vi "convertRateScanSettingsToString.vi"(8 "error in (no error)":errorcluster, 11 "Model in":refnum<class "Model.lvclass">) -> (0 "error out":errorcluster, 2 "Rate Scan Settings":string, 3 "Model out":refnum<class "Model.lvclass">)   [LabVIEW 2015, in "Model.lvclass"]
uses:
  Model.lvclass
  Model.lvclass/Model.ctl
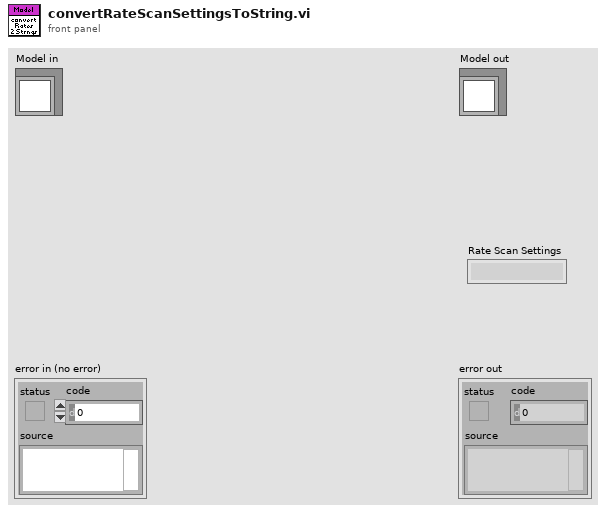
[diagram p1: front panel]
types:
  T1 = typedef "ILCCommon.lvlib/ILCConfiguration.lvlib/Scan Rates.ctl" = enum16{"50", "60", "100", "120", "200", "240", "300", "400", "480", "600", "1200", "2400", "4800"}
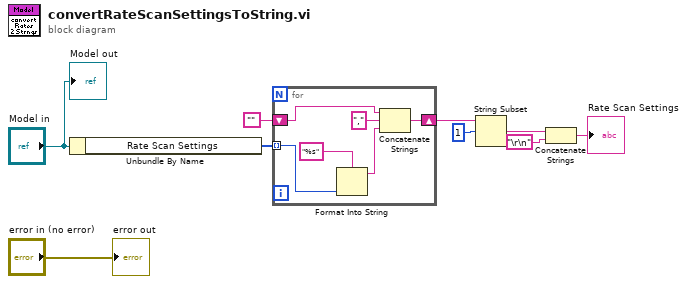
[diagram p0: block diagram]
diagram:
  n1 = Unbundle By Name("Model in") -> ("Rate Scan Settings"=w7:T1[])
  n2 = for {
    tunnel: w7 -> [w11] mode=indexing
    shift-right: [w15] -> w4
    shift-left: "" -> [w14]
    n3 = Format Into String(format string="%s", w11) -> (resulting string=w10:string)  [unwired: 2 in, 1 out]
    n4 = Concatenate Strings(w14, "," ("string"), w10) -> (w15:string)
  }
  n5 = String Subset(string=w4, offset (0)=1) -> (substring=w2:string)  [unwired: 1 in]
  n6 = Concatenate Strings(w2, "\r\n") -> (→"Rate Scan Settings":string)
  "error out" <- "error in (no error)"
  "Model out" <- "Model in"
